vi "Top Level VI.vi"() -> ()   [LabVIEW 2020]
doc: "This VI provides basic information about Top Level VI structure and basic functions of the VI Server Toolkit:\n1. Open/Close VI references.\n2. Set Controls, and\n3. Get Controls."
uses:
  VI Server Toolkit LV2013.lvlib
  VIS_Libraries/VI Server_Get Controls.llb/Recover DBL.vi
  VIS_Libraries/VI Server_Get Controls.llb/Recover STR.vi
  VI Server Libraries/VI Server_Set Controls.llb/Set 1D BOOL Control.vi
panel:
  in  "EXIT":bool
  in  "Tab.MAIN":enum32{"User Inputs", "Empty Page"}(tab)
  in  "Numeric.DBL":dbl
  in  "Numeric.DBL.Mirror":dbl
  in  "Numeric.DBL.String":string
  out "Error Out":errorcluster
  in  "Error In":errorcluster
  # "This VI demonstrates basic and yet fundamental features and functions of VI developed on the base of VI Server Toolkit.\n\nThe Top Level VI architecture can be described as:\n1. Open Control References.\n2. Core code.\n3. Close Controls references upon exit.\n\nThe fundamental functions of VI Server Tool Kit are:\n1. Get Control value and reference.\n2. Set Control Value.\n\nRun this VI.\n\nChange value of Numeric.DBL and observe the value of Numeric.DBL.Mirror control and Numeric.DBL.String control will be updated accordingly.\n\nChange the values of any controls and observe how this value will be passed to other two controls."
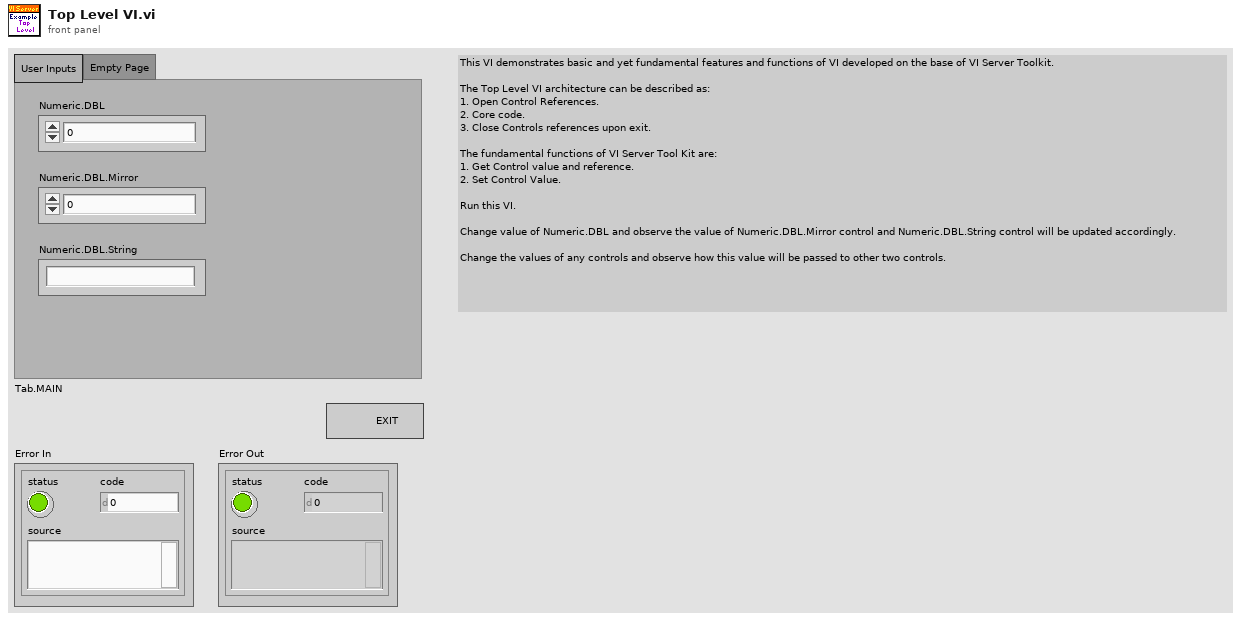
[diagram p1: front panel]
types:
  T1 = typedef "VI Server Toolkit LV2013.lvlib/VI Server Cluster.ctl" = cluster{"VI Ref":refnum<vi>, "Refs":refnum<vi>[], "Labels":string[]}
  T2 = typedef "VI Server_RefsCluster.ctl" = cluster{"Labels":string[], "Refs":refnum<vi>[], "VI Ref":refnum<vi>}
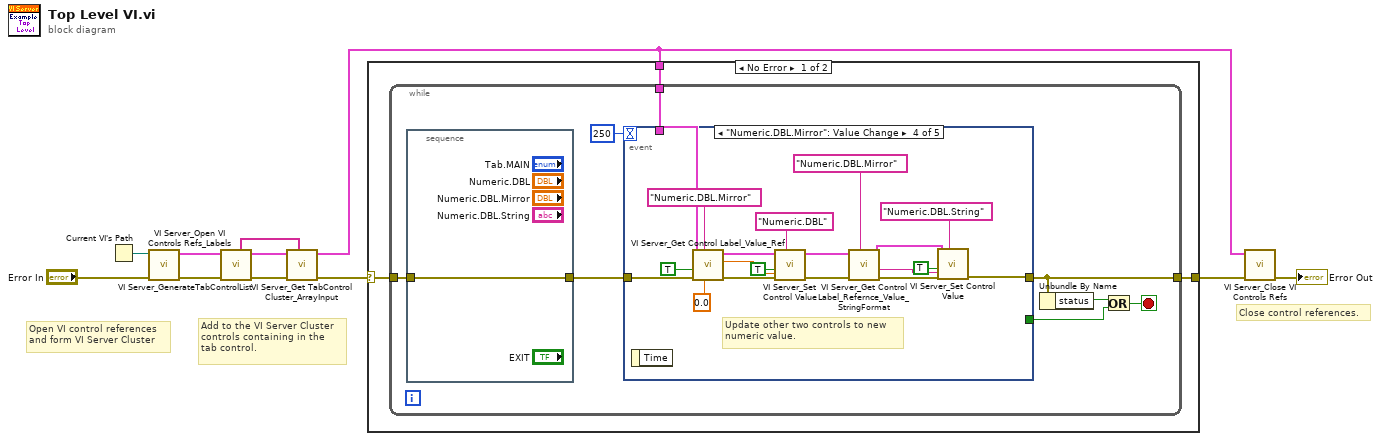
[diagram p0: block diagram]
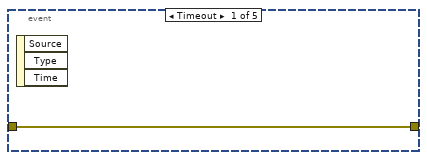
[diagram p2: hidden frame]
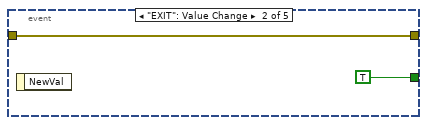
[diagram p3: hidden frame]
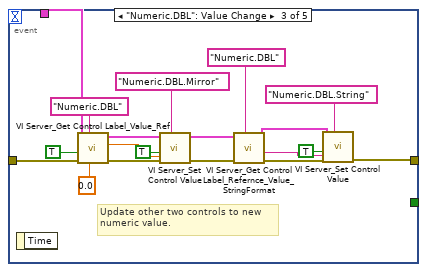
[diagram p4: hidden frame]
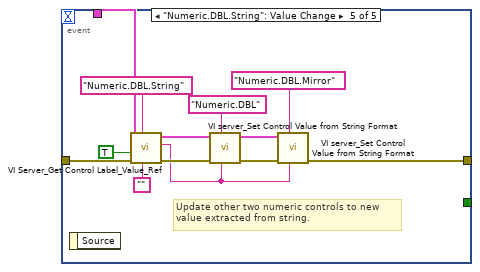
[diagram p5: hidden frame]
diagram:
  # "Close control references."
  # "Add to the VI Server Cluster\ncontrols containing in the\ntab control."
  # "Open VI control references\nand form VI Server Cluster"
  n1 = Current VI's Path() -> (path=w10:path)
  n2 = call "VI Server_Open VI Controls Refs_Labels.vi"("error in (no error)"="Error In", "Top Level VI Path"=w10) -> ("error out"=w9:errorcluster, "VI Server Cluster.OUT"=w8:T1)  [unwired: 8 in]
  n3 = call "VI Server_GenerateTabControlList.vi"("error in (no error)"=w9, "VI Server Cluster"=w8) -> ("error out"=w7:errorcluster, "VI Server Cluster.DUP"=w6:T2, "TabControls"=w5:string[])  [unwired: 7 in]
  n4 = call "VI Server_Get TabControl Cluster_ArrayInput.vi"("TabControl Labels[]"=w5, "error in"=w7, "VI Server Cluster"=w6) -> ("error out"=w4:errorcluster, "VI Server Cluster.OUT"=w1:T2)  [unwired: 7 in]
  n5 = case shown="No Error" w4 {
    selector: w4 -> [w14 w78]
    tunnel: [w13 w78] -> w3
    tunnel: w1 -> [w12 _]
    frame No Error {
      n6 = while {
        tunnel: w14 -> [w22]
        tunnel: [w19] -> w13
        tunnel: w12 -> [w15]
        stop <- w16 stop-if-true
        n7 = stacked-sequence {
          tunnel: w22 -> [w77]
          tunnel: [w77] -> w21
          frame #0 {
          }
        }
        n8 = event shown="[3] \"Numeric.DBL.Mirror\": Value Change" {
          selector: _ -> [_ _ _ _ _]
          dyn-events: _ -> [_ _ _ _ _]
          timeout: 250 -> [_ _ _ _ _]
          tunnel: w21 -> [w23 w25 w44 w63 w76]
          tunnel: [w23 w25 w26 w48 w64] -> w19
          tunnel: [_ TRUE _ _ _] -> w17
          tunnel: w15 -> [_ _ w42 w61 w74]
          event Timeout {
            n9 = event-data() -> ()  [unwired: 1 in, 3 out]
          }
          event "EXIT": Value Change {
            n10 = event-data() -> ()  [unwired: 1 in, 1 out]
          }
          event "Numeric.DBL": Value Change {
            # "Update other two controls to new\nnumeric value."
            n11 = event-data() -> ()  [unwired: 1 in, 1 out]
            n12 = call-poly "VI Server_Get Control Label_Value_Ref.vi"("Data Type"=0.0, "Label"="Numeric.DBL", "error in"=w44, "Single Instance (T)"=TRUE, "VI Server Cluster"=w42) -> ("error out"=w39:errorcluster, "Value"=w35:dbl, "VI Server Cluster.DUP"=w38:T1)  [unwired: 2 in, 2 out]
            n13 = call-poly "VI Server_Set Control Value.vi"("New Value"=w35, "Label"="Numeric.DBL.Mirror", "error in"=w39, "Single Instance (T)"=TRUE, "VI Server Cluster"=w38) -> ("error out"=w34:errorcluster, "VI Server Cluster.DUP"=w33:T2)  [unwired: 4 in, 1 out]
            n14 = call <vilib>:"VI Server_Get Control Label_Refernce_Value_StringFormat.vi"("Label"="Numeric.DBL", "error in (no error)"=w34, "VI Server Cluster"=w33) -> ("error out"=w31:errorcluster, "ControlValue(StringFormat)"=w27:string, "VI Server Cluster.DUP"=w29:T1)  [unwired: 6 in]
            n15 = call-poly "VI Server_Set Control Value.vi"("New Value"=w27, "Label"="Numeric.DBL.String", "error in"=w31, "Single Instance (T)"=TRUE, "VI Server Cluster"=w29) -> ("error out"=w26:errorcluster)  [unwired: 4 in, 2 out]
          }
          event "Numeric.DBL.Mirror": Value Change {
            # "Update other two controls to new\nnumeric value."
            n16 = event-data() -> ()  [unwired: 1 in, 1 out]
            n17 = call-poly "VI Server_Get Control Label_Value_Ref.vi"("Data Type"=0.0, "Label"="Numeric.DBL.Mirror", "error in"=w63, "Single Instance (T)"=TRUE, "VI Server Cluster"=w61) -> ("error out"=w59:errorcluster, "Value"=w56:dbl, "VI Server Cluster.DUP"=w58:T1)  [unwired: 2 in, 2 out]
            n18 = call-poly "VI Server_Set Control Value.vi"("New Value"=w56, "Label"="Numeric.DBL", "error in"=w59, "Single Instance (T)"=TRUE, "VI Server Cluster"=w58) -> ("error out"=w55:errorcluster, "VI Server Cluster.DUP"=w54:T2)  [unwired: 4 in, 1 out]
            n19 = call <vilib>:"VI Server_Get Control Label_Refernce_Value_StringFormat.vi"("Label"="Numeric.DBL.Mirror", "error in (no error)"=w55, "VI Server Cluster"=w54) -> ("error out"=w53:errorcluster, "ControlValue(StringFormat)"=w49:string, "VI Server Cluster.DUP"=w51:T1)  [unwired: 6 in]
            n20 = call-poly "VI Server_Set Control Value.vi"("New Value"=w49, "Label"="Numeric.DBL.String", "error in"=w53, "Single Instance (T)"=TRUE, "VI Server Cluster"=w51) -> ("error out"=w48:errorcluster)  [unwired: 4 in, 2 out]
          }
          event "Numeric.DBL.String": Value Change {
            # "Update other two numeric controls to new\nvalue extracted from string."
            n21 = event-data() -> ()  [unwired: 1 in, 1 out]
            n22 = call-poly "VI Server_Get Control Label_Value_Ref.vi"("Data Type"="", "Label"="Numeric.DBL.String", "error in"=w76, "Single Instance (T)"=TRUE, "VI Server Cluster"=w74) -> ("error out"=w71:errorcluster, "Value"=w65:string, "VI Server Cluster.DUP"=w70:T1)  [unwired: 2 in, 2 out]
            n23 = call "VI server_Set Control Value from String Format.vi"("Value.STR"=w65, "Label"="Numeric.DBL", "error in (no error)"=w71, "VI Server Cluster"=w70) -> ("error out"=w68:errorcluster, "VI Server Cluster.DUP"=w67:T2)  [unwired: 5 in, 1 out]
            n24 = call "VI server_Set Control Value from String Format.vi"("Value.STR"=w65, "Label"="Numeric.DBL.Mirror", "error in (no error)"=w68, "VI Server Cluster"=w67) -> ("error out"=w64:errorcluster)  [unwired: 5 in, 2 out]
          }
        }
        n25 = Unbundle By Name(w19) -> ("status"=w18:bool)
        n26 = Or(x=w18, y=w17) -> (x .or. y?=w16:bool)
      }
    }
    frame Error {
    }
  }
  n27 = call "VI Server_Close VI Controls Refs.vi"("error in (no error)"=w3, "VI Server Cluster"=w1) -> ("error out"=→"Error Out":errorcluster)  [unwired: 9 in]
